vi "demo_This Month in LabVIEW (TMiLV).vi"(11 "Stop Demo":refnum<user-event>) -> ()   [LabVIEW 2020]
panel:
  # "TMiLV - This Month in LabVIEW podcast (aka the worlds worst acronym)\n\nNews and opinion once a month, all about making stuff with LabVIEW\nLed by Steve Watts and Nancy Henson, dive into discussions high and low and as a minimum...be entertained.\nhttps://www.youtube.com/@ThisMonthInLabVIEW/"
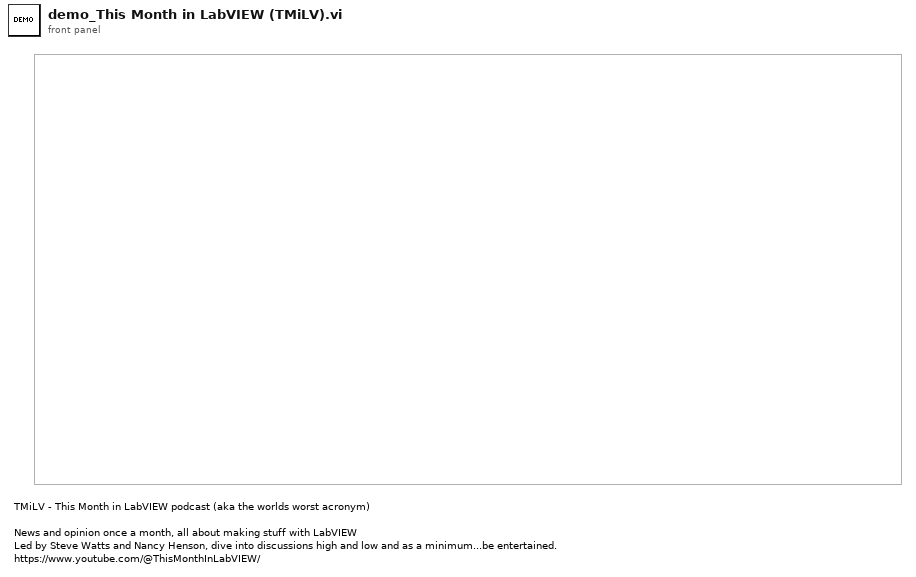
[diagram p1: front panel]
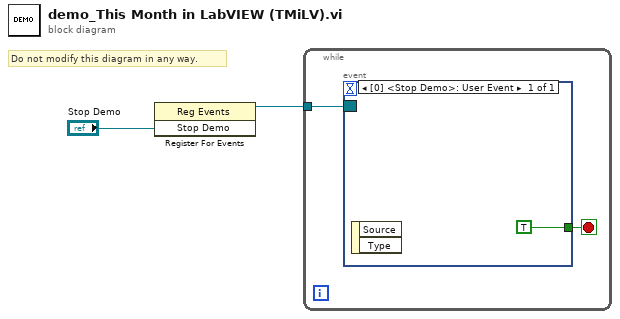
[diagram p0: block diagram]
diagram:
  # "Do not modify this diagram in any way."
  n1 = register-events("Stop Demo") -> (reference out=w1:refnum<event-registration>)  [unwired: 2 in, 1 out]
  n2 = while {
    tunnel: w1 -> [w4]
    stop <- w3 stop-if-true
    n3 = event shown="[0] <Stop Demo>: User Event" {
      selector: w4 -> [_]
      dyn-events: _ -> [_]
      timeout: _ -> [_]
      tunnel: [TRUE] -> w3
      event User Event {
        n4 = event-data() -> ()  [unwired: 1 in, 2 out]
      }
    }
  }
